vi "Autenticacion.vi"(2 "Operario":string, 3 "TieneAcceso?":bool) -> (0 "AccesoPermitido":bool, 1 "IntentosUsados":dbl)   [LabVIEW 2017]
uses:
  Control/Enum_Autenticacion.ctl
panel:
  out "usedToVerificateRead2Times":bool
  out "Mensaje de error":string
  out "Elementos":dbl[](array[numeric])
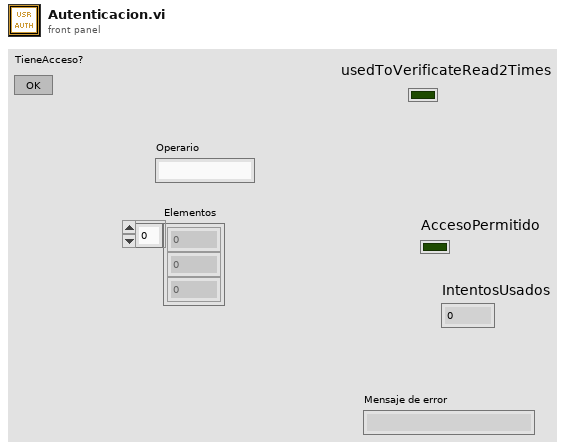
[diagram p1: front panel]
types:
  T1 = typedef "Enum_Autenticacion.ctl" = enum16{"Default", "Read", "Write", "DeleteAll", "Restart", "Verification", "Error", "Stop"}
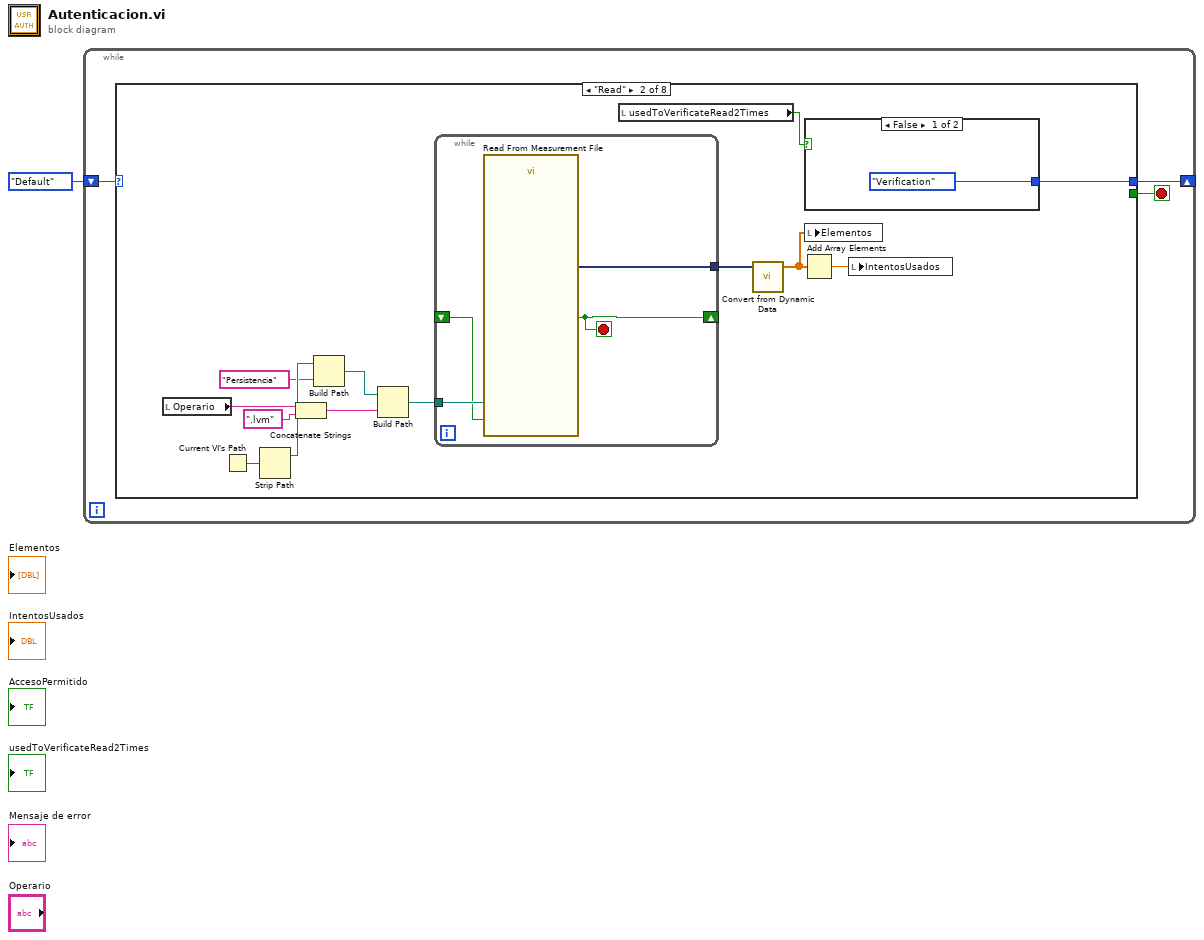
[diagram p0: block diagram]
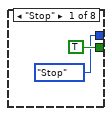
[diagram p2: hidden frame]
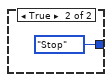
[diagram p3: hidden frame]
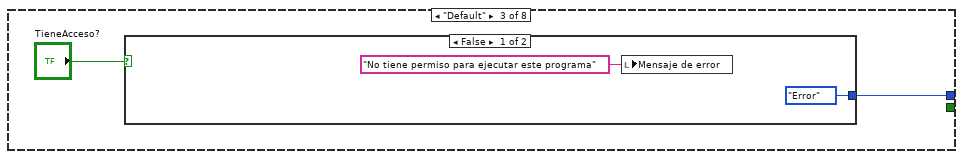
[diagram p4: hidden frame]
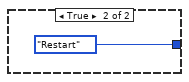
[diagram p5: hidden frame]
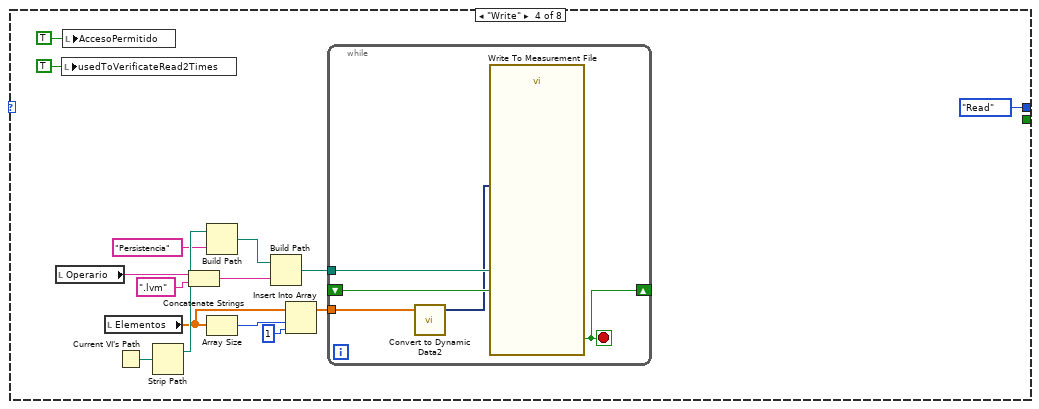
[diagram p6: hidden frame]
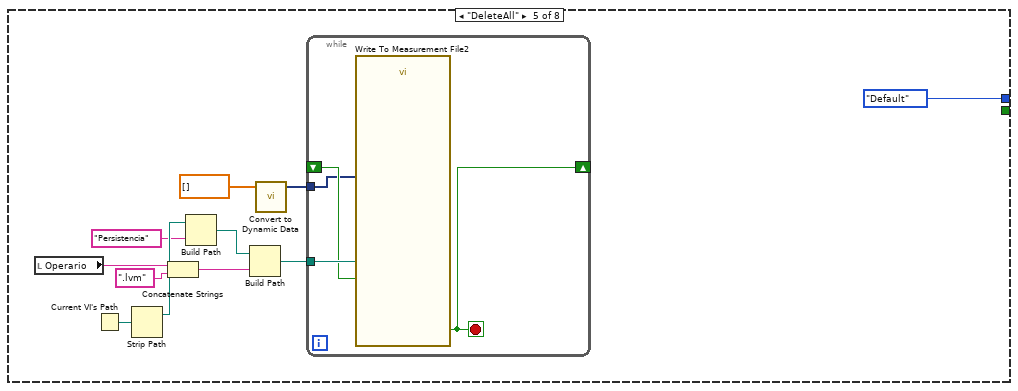
[diagram p7: hidden frame]
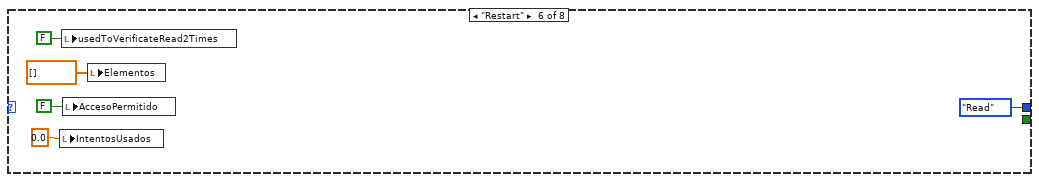
[diagram p8: hidden frame]
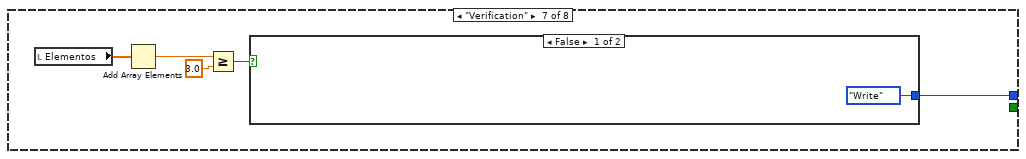
[diagram p9: hidden frame]
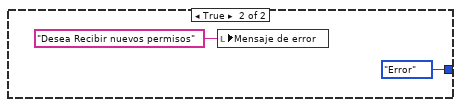
[diagram p10: hidden frame]
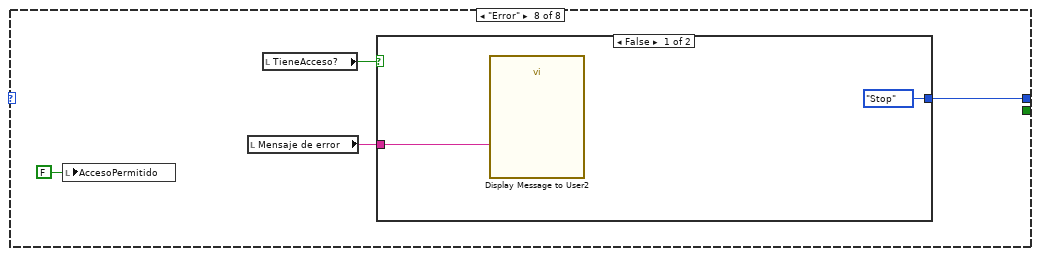
[diagram p11: hidden frame]
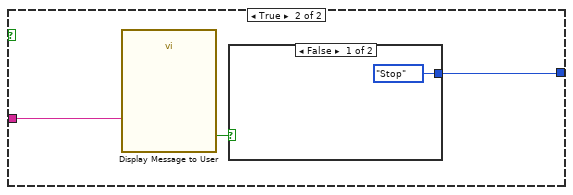
[diagram p12: hidden frame]
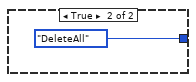
[diagram p13: hidden frame]
diagram:
  n1 = while {
    shift-right: [w3] -> _
    shift-left: Enum_Autenticacion."Default" -> [w4]
    stop <- w2 stop-if-true
    n2 = case shown="\"Read\"" w4 {
      tunnel: [TRUE _ _ _ _ _ _ _] -> w2
      tunnel: [Enum_Autenticacion."Stop" w10 w26 Enum_Autenticacion."Read" Enum_Autenticacion."Default" Enum_Autenticacion."Read" w72 w81] -> w3
      frame "Stop" {
      }
      frame "Read" {
        n3 = local read "Operario"() -> (w11:string)
        n4 = Current VI's Path() -> (path=w15:path)
        n5 = Strip Path(path=w15) -> (stripped path=w17:path)  [unwired: 1 out]
        n6 = Concatenate Strings(w11, ".lvm" ("string")) -> (w13:string)
        n7 = Build Path(base path=w17, name or relative path="Persistencia") -> (appended path=w16:path)
        n8 = Build Path(base path=w16, name or relative path=w13) -> (appended path=w18:path)
        n9 = while {
          tunnel: w18 -> [w25]
          tunnel: [w24] -> w12
          shift-right: [w22] -> _
          shift-left: _ -> [w23]
          stop <- w22 stop-if-true
          n10 = call "Read From Measurement File"("Filename"=w25, "Reset"=w23) -> ("Signals"=w24:dynamicdata, "EOF?"=w22:bool)  [unwired: 4 in, 4 out]
        }
        n11 = local read "usedToVerificateRead2Times"() -> (w9:bool)
        n12 = call "Convert from Dynamic Data"("Dynamic Data Type"=w12) -> ("Array"=w8:dbl[])  [unwired: 3 in]
        n13 = Add Array Elements(numeric array=w8) -> (sum=w7:dbl)
        n14 = case shown="False" w9 {
          tunnel: [Enum_Autenticacion."Verification" Enum_Autenticacion."Stop"] -> w10
          frame False {
          }
          frame True {
          }
        }
        n15 = local write "Elementos"(w8) -> ()
        n16 = local write "IntentosUsados"(w7) -> ()
      }
      frame "Default" {
        n17 = case shown="False" "TieneAcceso?" {
          tunnel: [Enum_Autenticacion."Error" Enum_Autenticacion."Restart"] -> w26
          frame False {
            n18 = local write "Mensaje de error"("No tiene permiso para ejecutar este programa" ("Mensaje de error")) -> ()
          }
          frame True {
          }
        }
      }
      frame "Write" {
        n19 = local read "Operario"() -> (w38:string)
        n20 = local write "usedToVerificateRead2Times"(TRUE ("Boolean")) -> ()
        n21 = local write "AccesoPermitido"(TRUE ("Boolean")) -> ()
        n22 = local read "Elementos"() -> (w35:dbl[])
        n23 = Current VI's Path() -> (path=w40:path)
        n24 = Strip Path(path=w40) -> (stripped path=w45:path)  [unwired: 1 out]
        n25 = Concatenate Strings(w38, ".lvm" ("string")) -> (w42:string)
        n26 = Build Path(base path=w45, name or relative path="Persistencia") -> (appended path=w44:path)
        n27 = Array Size(array=w35) -> (size(s)=w36:i32)
        n28 = Build Path(base path=w44, name or relative path=w42) -> (appended path=w39:path)
        n29 = Insert Into Array(array=w35, index=w36, new element=1) -> (w33:dbl[])
        n30 = while {
          tunnel: w39 -> [w50]
          shift-right: [w49] -> _
          shift-left: _ -> [w48]
          tunnel: w33 -> [w47]
          stop <- w49 stop-if-true
          n31 = call "Convert to Dynamic Data2"("Array"=w47) -> ("Dynamic Data Type"=w46:dynamicdata)  [unwired: 3 in]
          n32 = call "Write To Measurement File"("Signals"=w46, "Reset"=w48, "Filename"=w50) -> ("Saving Data"=w49:bool)  [unwired: 14 in, 2 out]
        }
      }
      frame "DeleteAll" {
        n33 = local read "Operario"() -> (w54:string)
        n34 = Current VI's Path() -> (path=w56:path)
        n35 = Strip Path(path=w56) -> (stripped path=w61:path)  [unwired: 1 out]
        n36 = Concatenate Strings(w54, ".lvm" ("string")) -> (w58:string)
        n37 = Build Path(base path=w61, name or relative path="Persistencia") -> (appended path=w60:path)
        n38 = Build Path(base path=w60, name or relative path=w58) -> (appended path=w55:path)
        n39 = call "Convert to Dynamic Data"("Array"=dbl[] []) -> ("Dynamic Data Type"=w52:dynamicdata)  [unwired: 3 in]
        n40 = while {
          tunnel: w55 -> [w65]
          shift-right: [w64] -> _
          shift-left: _ -> [w63]
          tunnel: w52 -> [w62]
          stop <- w64 stop-if-true
          n41 = call "Write To Measurement File2"("Signals"=w62, "Reset"=w63, "Filename"=w65) -> ("Saving Data"=w64:bool)  [unwired: 14 in, 2 out]
        }
      }
      frame "Restart" {
        n42 = local write "IntentosUsados"(0.0 ("IntentosUsados")) -> ()
        n43 = local write "usedToVerificateRead2Times"(FALSE ("Boolean")) -> ()
        n44 = local write "AccesoPermitido"(FALSE ("AccesoPermitido")) -> ()
        n45 = local write "Elementos"(dbl[] [] ("Elementos")) -> ()
      }
      frame "Verification" {
        n46 = local read "Elementos"() -> (w75:dbl[])
        n47 = Add Array Elements(numeric array=w75) -> (sum=w71:dbl)
        n48 = Greater Or Equal?(x=w71, y=3.0) -> (x >= y?=w73:bool)
        n49 = case shown="False" w73 {
          tunnel: [Enum_Autenticacion."Write" Enum_Autenticacion."Error"] -> w72
          frame False {
          }
          frame True {
            n50 = local write "Mensaje de error"("Desea Recibir nuevos permisos" ("Mensaje de error")) -> ()
          }
        }
      }
      frame "Error" {
        n51 = local write "AccesoPermitido"(FALSE ("AccesoPermitido")) -> ()
        n52 = local read "Mensaje de error"() -> (w82:string)
        n53 = local read "TieneAcceso?"() -> (w79:bool)
        n54 = case shown="False" w79 {
          tunnel: w82 -> [w84 w87]
          tunnel: [Enum_Autenticacion."Stop" w85] -> w81
          frame False {
            n55 = call "Display Message to User2"("Message"=w84) -> ()  [unwired: 9 in, 2 out]
          }
          frame True {
            n56 = call "Display Message to User"("Message"=w87) -> ("Si"=w86:bool)  [unwired: 9 in, 1 out]
            n57 = case shown="False" w86 {
              tunnel: [Enum_Autenticacion."Stop" Enum_Autenticacion."DeleteAll"] -> w85
              frame False {
              }
              frame True {
              }
            }
          }
        }
      }
    }
  }
